vi "Switch Configuration.vi"(8 "error in (no error)":errorcluster, 11 "Node Ptr":T2 format="%.0x") -> (0 "error out":errorcluster)   [LabVIEW 2015, in "DMM-SWITCH-ScanList System Explorer.lvlib"]
uses:
  DMM-SWITCH-ScanList System Explorer.lvlib
  <vilib>/NI Veristand/Custom Device API/Custom Device Item Ref.ctl
  <instrlib>/niSwitch/niSwitch.LLB/niSwitch Topologies.ctl
  Configuration Controls/Switch Config VI UI Data.ctl
  Configuration Controls/Switch Config VI UI Ctrl Values.ctl
  Configuration Controls/Switch Config VI UI Ctrl References.ctl
  <vilib>/NI Veristand/Custom Device API/Custom Device API.lvlib
panel:
  in  "Switch Resource Name":string
  out "Generated Scan List String":string
  in  "Scan List String":string
  in  "Scan List Automatic/Manual":bool=TRUE
  in  "Connect ab0":bool
  in  "Topology Names":T1="2503/2-Wire 24x1 Mux" caption="topology name"
  in  "Save":bool
  in  "Channels":i32[](listbox)
  in  "Switch Model":string(combo)
  in  "Topology":string(combo)
  in  "Remove All":bool
  in  "Add All":bool
  in  "Selectable Channels":i32[](listbox)
  in  "Remove Channels":bool
  in  "Add Channels":bool
  in  "Header":cluster{"Section Name":string}={"Section Name"="Custom Device Item Settings"}
  in  "Description":string
  in  "Name":string
  in  "Update Scan List":bool
  # "Scan List String"
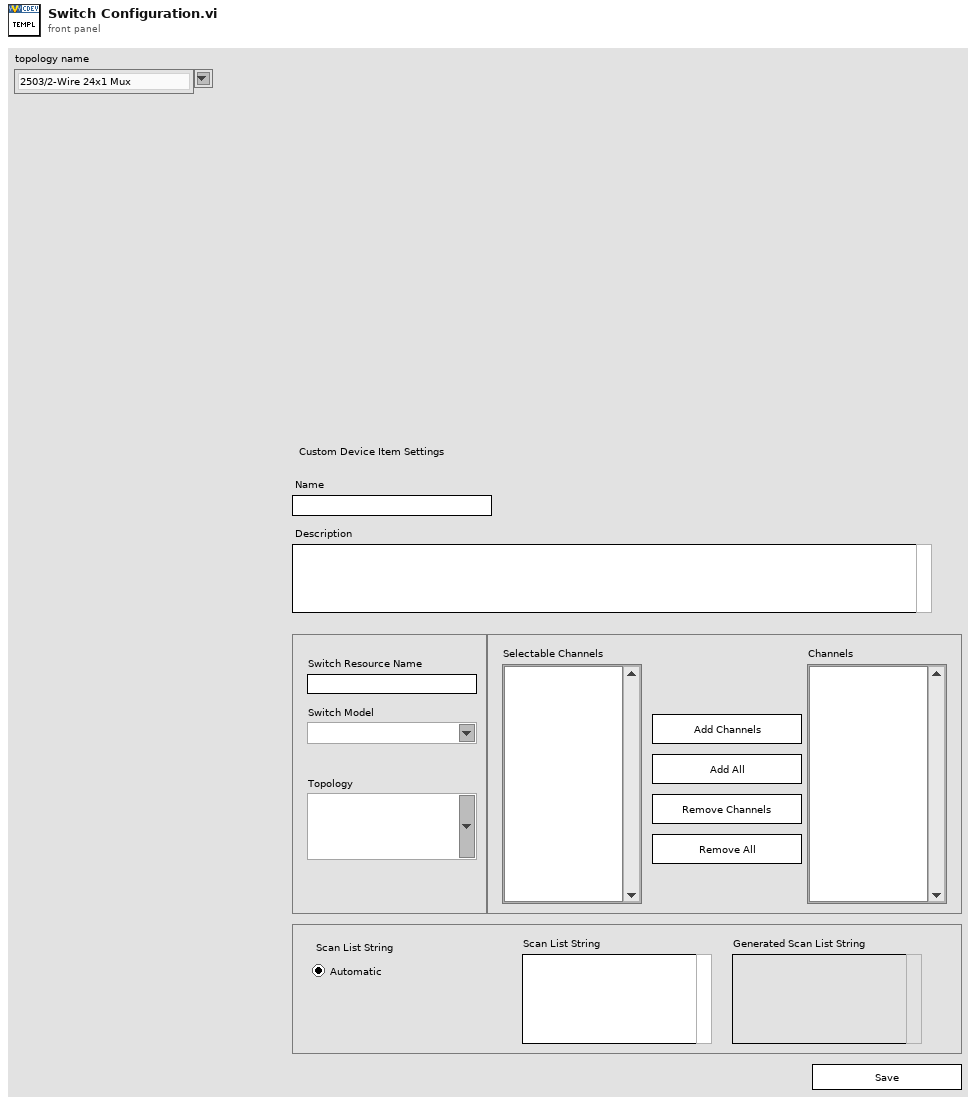
[diagram p1: front panel]
types:
  T1 = typedef "niSwitch Topologies.ctl" = string
  T2 = typedef "Custom Device API.lvlib/Custom Device Item Ref.ctl" = u64
  T3 = typedef "DMM-SWITCH-ScanList System Explorer.lvlib/Switch Config VI UI Data.ctl" = cluster{"Ctrl Values":T4, "Crtl Refs":T5, "Switch Config Page Item Ref":T2, "Mux List":string[]}
  T4 = typedef "DMM-SWITCH-ScanList System Explorer.lvlib/Switch Config VI UI Ctrl Values.ctl" = cluster{"Switch Resource Name":string, "Switch Model":string, "Topology":string, "Selectable Channels":i32[], "Channels":i32[], "Scan List String Mode":bool, "Connect ab0":bool, "Generated Scan List String":string, "Scan List String":string}
  T5 = typedef "DMM-SWITCH-ScanList System Explorer.lvlib/Switch Config VI UI Ctrl References.ctl" = cluster{"Update Scan List":refnum<vi>, "Generated Scan List String":refnum<vi>, "Scan List String":refnum<vi>, "Connect ab0":refnum<vi>, "Selectable Channels":refnum<vi>, "Channels":refnum<vi>, "Topology":refnum<vi>, "Switch Model":refnum<vi>, "Topology Names":refnum<vi>}
  T6 = typedef "Custom Device API.lvlib/Custom Device Item Info.ctl" = cluster{"Name":string, "Is Channel":bool, "GUID":string, "Is Waveform":bool}
  T7 = typedef "Custom Device API.lvlib/Custom Device Commands.ctl" = enum16{"Default", "Item renamed", "Shutdown", "Dynamic button pressed"}
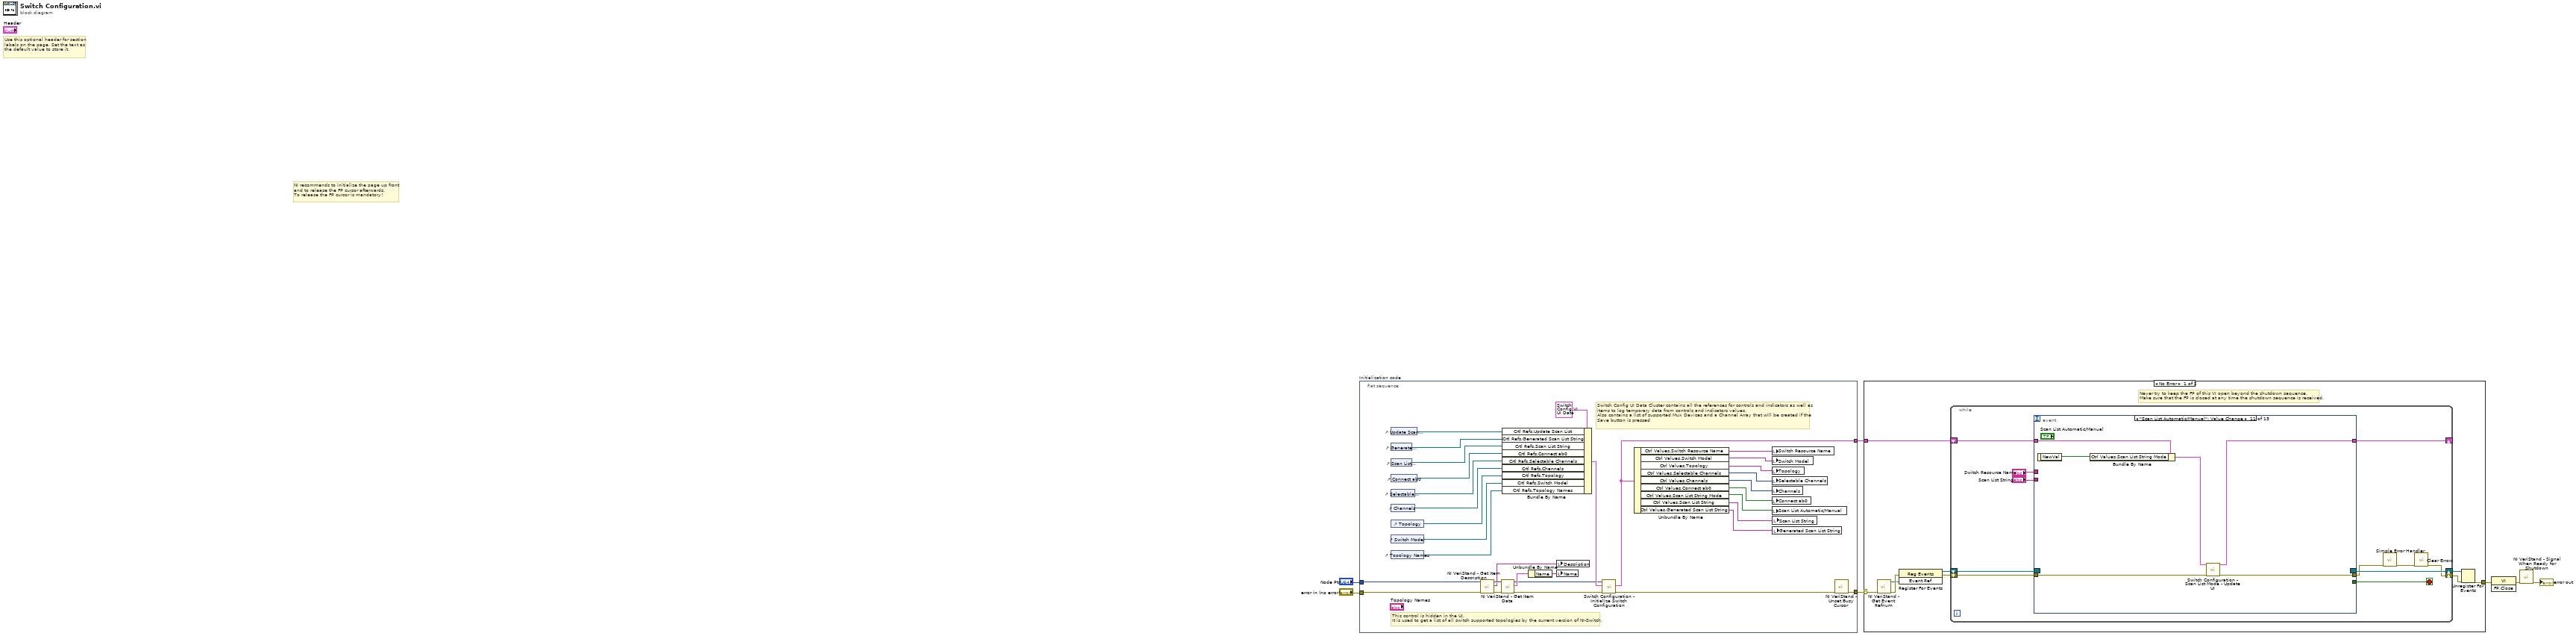
[diagram p0: block diagram]
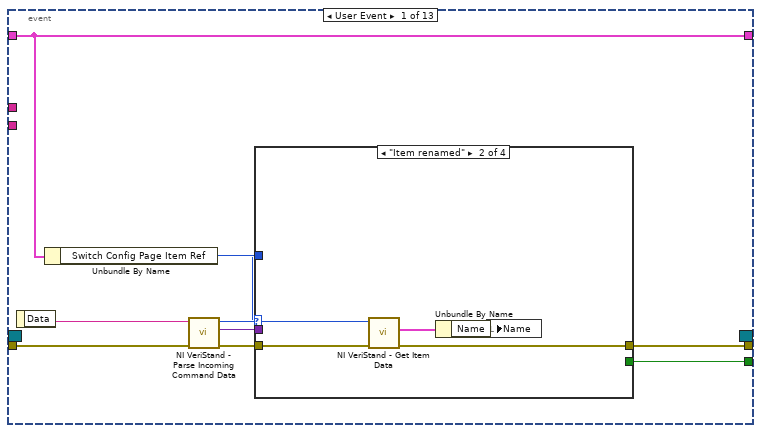
[diagram p2: hidden frame]
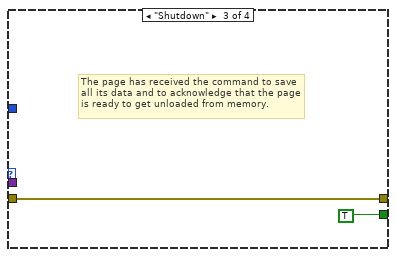
[diagram p4: hidden frame]
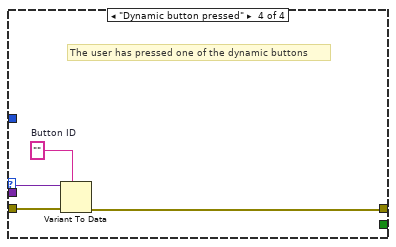
[diagram p5: hidden frame]
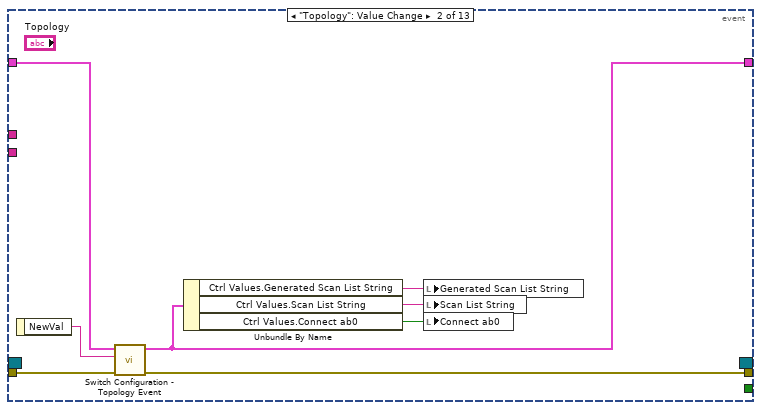
[diagram p6: hidden frame]
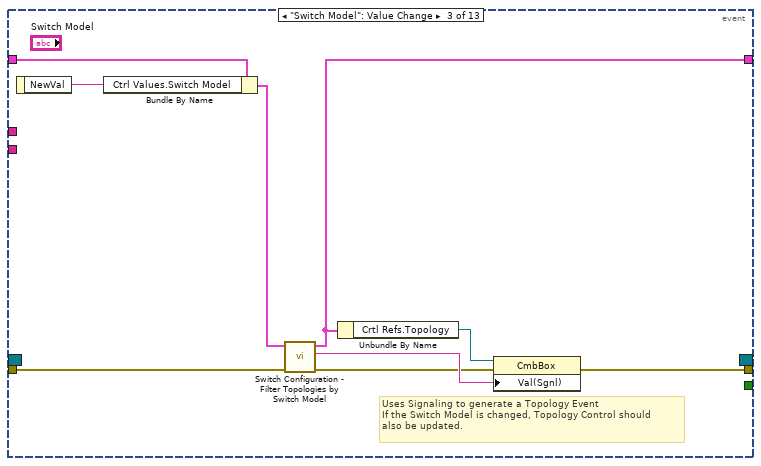
[diagram p7: hidden frame]
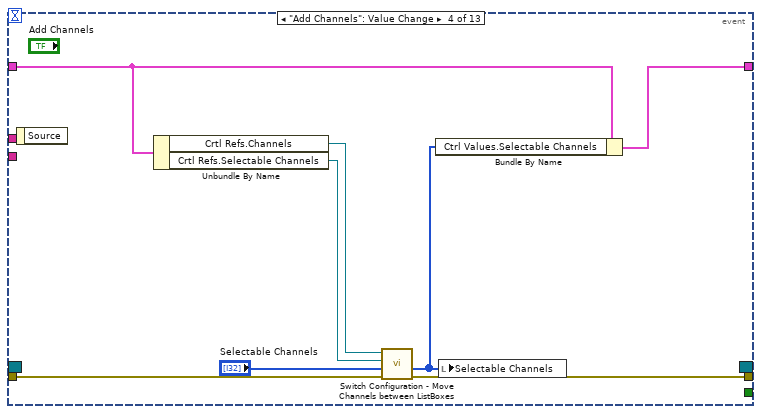
[diagram p8: hidden frame]
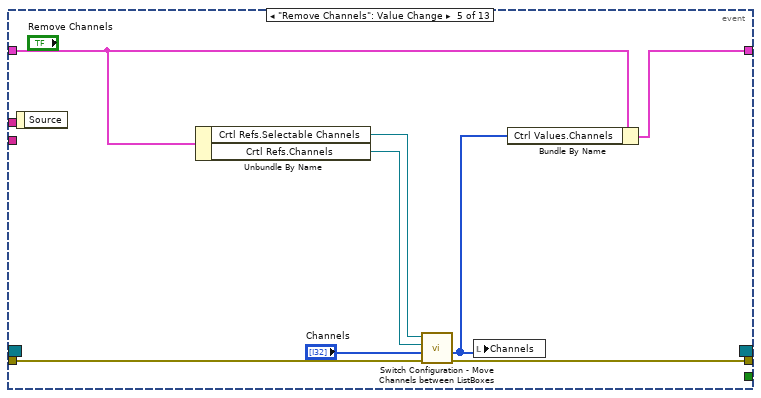
[diagram p9: hidden frame]
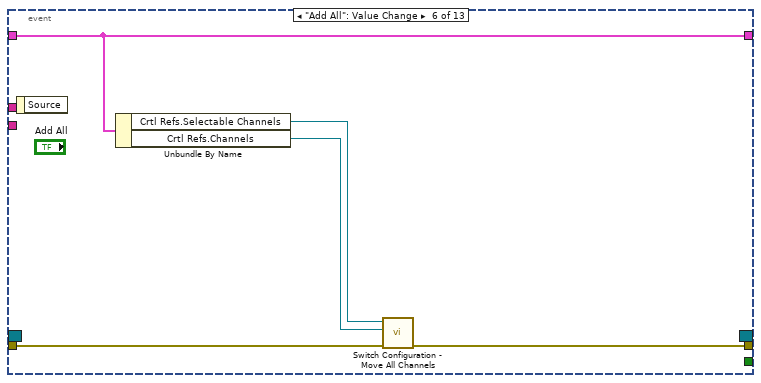
[diagram p10: hidden frame]
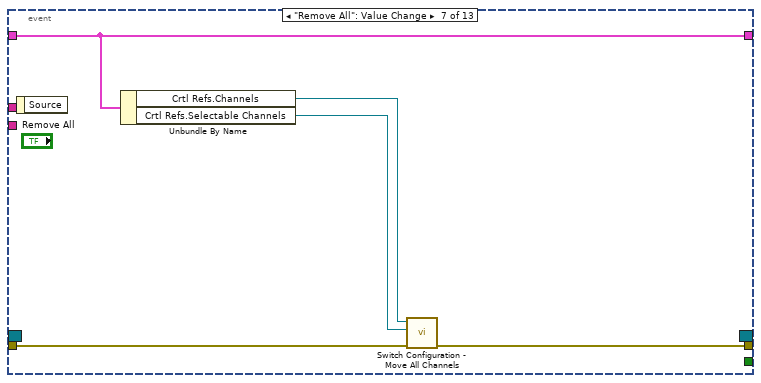
[diagram p11: hidden frame]
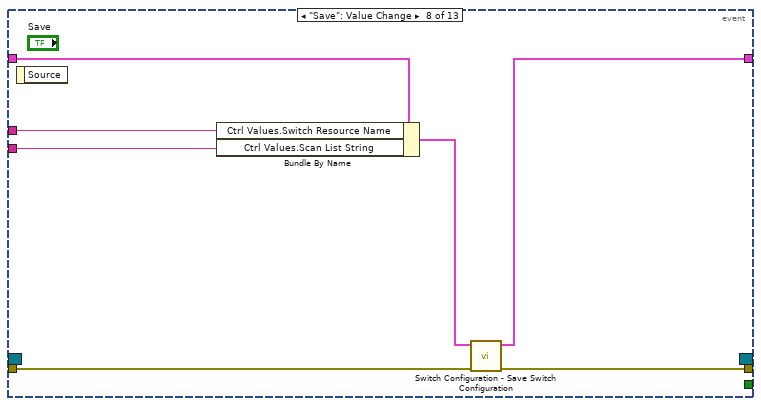
[diagram p12: hidden frame]
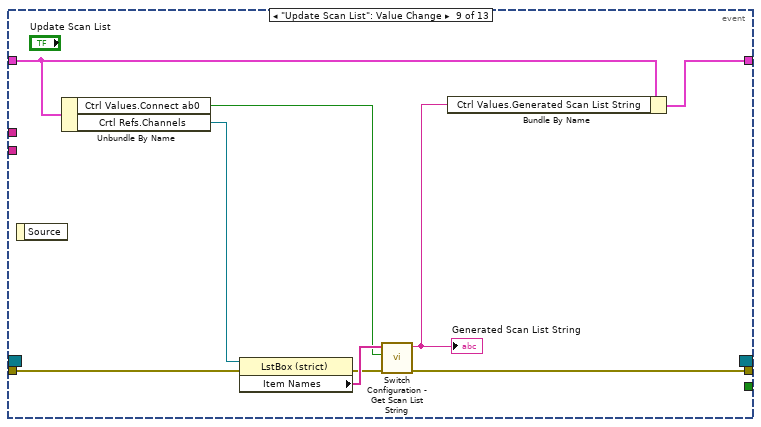
[diagram p13: hidden frame]
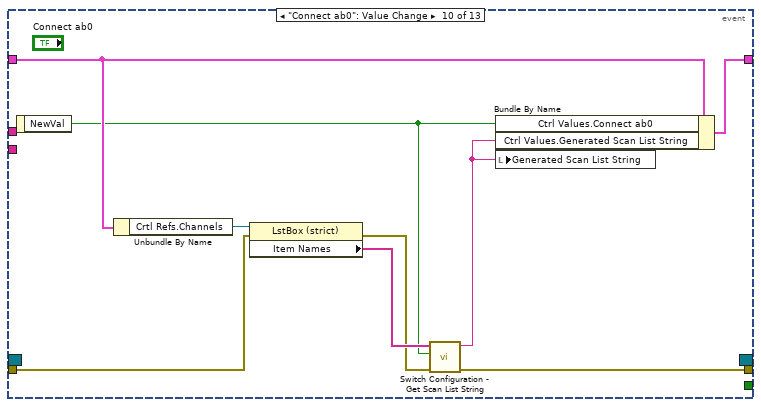
[diagram p14: hidden frame]
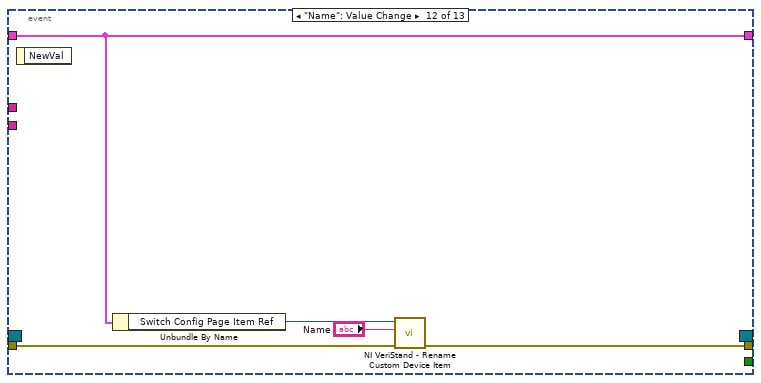
[diagram p15: hidden frame]
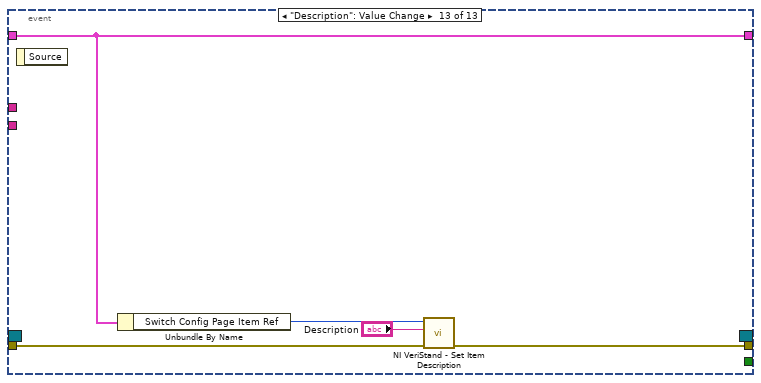
[diagram p16: hidden frame]
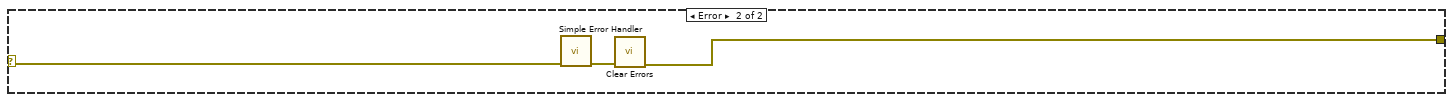
[diagram p17: hidden frame]
diagram:
  # "Use this optional header for section labels on the page. Set the text as the default value to store it."
  # "NI recommends to initialize the page up front\nand to release the FP cursor afterwards.\nTo release the FP cursor is mandatory!"
  n1 = flat-sequence "Initialization code" {
    tunnel: "error in (no error)" -> [w38]
    tunnel: "Node Ptr" -> [w37]
    tunnel: [w20] -> w2
    tunnel: [w10] -> w1
    frame #0 {
      # "This control is hidden in the UI. \nIt is used to get a list of all switch supported topologies by the current version of NI-Switch."
      # "Switch Config UI Data Cluster contains all the references for controls and indicators as well as\nitems to log temporary data from controls and indicators values.\nAlso contains a list of supported Mux Devices and a Channel Array that will be created if the\nSave button is pressed"
      n2 = control-ref of="Update Scan List"() -> (w28:refnum<vi>)
      n3 = control-ref of="Generated Scan List String"() -> (w29:refnum<vi>)
      n4 = control-ref of="Scan List String"() -> (w30:refnum<vi>)
      n5 = control-ref of="Connect ab0"() -> (w31:refnum<vi>)
      n6 = control-ref of="Selectable Channels"() -> (w22:refnum<vi>)
      n7 = control-ref of="Channels"() -> (w23:refnum<vi>)
      n8 = control-ref of="Topology"() -> (w24:refnum<vi>)
      n9 = control-ref of="Switch Model"() -> (w27:refnum<vi>)
      n10 = control-ref of="Topology Names"() -> (w26:refnum<vi>)
      n11 = call <vilib>:"NI VeriStand - Get Item Description.vi"("error in (no error)"=w38, "Item Ref in"=w37) -> ("error out"=w35:errorcluster, "Description"=w36:string, "Item Ref out"=w39:T2)  [unwired: 7 out]
      n12 = call <vilib>:"NI VeriStand - Get Item Data.vi"("error in (no error)"=w35, "Item Ref in"=w39) -> ("error out"=w32:errorcluster, "Item Info"=w34:T6, "Item Ref out"=w9:T2)  [unwired: 7 out]
      n13 = Bundle By Name(cluster=T3 {"Ctrl Values"={"Switch Resource Name"="", "Switch Model"="", "Topology"="", "Selectable Channels"=[], "Channels"=[], "Scan List String Mode"=FALSE, "Connect ab0"=FALSE, "Generated Scan List String"="", "Scan List String"=""}, "Crtl Refs"={"Update Scan List"=refnum, "Generated Scan List String"=refnum, "Scan List String"=refnum, "Connect ab0"=refnum, "Selectable Channels"=refnum, "Channels"=refnum, "Topology"=refnum, "Switch Model"=refnum, "Topology Names"=refnum}, "Switch Config Page Item Ref"=0, "Mux List"=[]} ("Switch Config UI Data"), "Crtl Refs.Update Scan List"=w28, "Crtl Refs.Generated Scan List String"=w29, "Crtl Refs.Scan List String"=w30, "Crtl Refs.Connect ab0"=w31, "Crtl Refs.Selectable Channels"=w22, "Crtl Refs.Channels"=w23, "Crtl Refs.Topology"=w24, "Crtl Refs.Switch Model"=w27, "Crtl Refs.Topology Names"=w26) -> (w21:T3)
      n14 = Unbundle By Name(w34) -> ("Name"=w33:string)
      n15 = local write "Description"(w36) -> ()
      n16 = local write "Name"(w33) -> ()
      n17 = call "Switch Configuration - Initialize Switch Configuration.vi"("error in (no error)"=w32, "Switch Config UI Data in"=w21, "Item Ref in"=w9) -> ("error out"=w8:errorcluster, "Switch Config UI Data out"=w20:T3)  [unwired: 7 in]
      n18 = Unbundle By Name(w20) -> ("Ctrl Values.Switch Resource Name"=w19:string, "Ctrl Values.Switch Model"=w18:string, "Ctrl Values.Topology"=w17:string, "Ctrl Values.Selectable Channels"=w16:i32[], "Ctrl Values.Channels"=w15:i32[], "Ctrl Values.Connect ab0"=w14:bool, "Ctrl Values.Scan List String Mode"=w13:bool, "Ctrl Values.Scan List String"=w12:string, "Ctrl Values.Generated Scan List String"=w11:string)
      n19 = local write "Switch Resource Name"(w19) -> ()
      n20 = local write "Switch Model"(w18) -> ()
      n21 = local write "Topology"(w17) -> ()
      n22 = local write "Selectable Channels"(w16) -> ()
      n23 = local write "Channels"(w15) -> ()
      n24 = local write "Connect ab0"(w14) -> ()
      n25 = local write "Scan List Automatic/Manual"(w13) -> ()
      n26 = local write "Scan List String"(w12) -> ()
      n27 = local write "Generated Scan List String"(w11) -> ()
      n28 = call <vilib>:"NI VeriStand - Unset Busy Cursor.vi"("error in (no error)"=w8) -> ("error out"=w10:errorcluster)  [unwired: 10 out]
    }
  }
  n29 = case shown="No Error" w1 {
    selector: w1 -> [w41 w167]
    tunnel: [w45 w165] -> w7
    tunnel: w2 -> [w40 _]
    frame No Error {
      # "Never try to keep the FP of this VI open beyond the shutdown sequence.\nMake sure that the FP is closed at any time the shutdown sequence is received."
      n30 = call <vilib>:"NI VeriStand - Get Event Refnum.vi"("error in (no error)"=w41) -> ("error out"=w48:errorcluster, "Event Ref"=w44:refnum<user-event>)  [unwired: 9 out]
      n31 = register-events(error in=w48, w44) -> (reference out=w42:refnum<event-registration>, error out=w43:errorcluster)  [unwired: 1 in]
      n32 = while {
        shift-right: [w55] -> w46
        shift-left: w43 -> [w58]
        shift-right: [w59] -> w47
        shift-left: w42 -> [w57]
        shift-right: [w53] -> _
        shift-left: w40 -> [w54]
        stop <- w56 stop-if-true
        n33 = event shown="[10] \"Scan List Automatic/Manual\": Value Change" {
          selector: w57 -> [_ _ _ _ _ _ _ _ _ _ _ _ _]
          dyn-events: [_ _ _ _ _ _ _ _ _ _ _ _ _] -> w59
          timeout: _ -> [_ _ _ _ _ _ _ _ _ _ _ _ _]
          tunnel: w58 -> [w68 w88 w92 w105 w113 w118 w123 w129 w139 w148 w154 w159 w164]
          tunnel: [w64 _ _ _ _ _ _ _ _ _ _ _ _] -> w56
          tunnel: [w63 w87 w95 w103 w111 w117 w122 w130 w136 w145 w153 w158 w163] -> w52
          tunnel: w54 -> [w61 w86 w91 w100 w107 w114 w119 w128 w134 w142 w151 w156 w161]
          tunnel: [w61 w85 w89 w98 w106 w114 w119 w124 w132 w141 w149 w156 w161] -> w53
          tunnel: "Switch Resource Name" -> [_ _ _ _ _ _ _ w127 _ _ _ _ _]
          tunnel: "Scan List String" -> [_ _ _ _ _ _ _ w126 _ _ _ _ _]
          event User Event {
            n34 = event-data() -> ("Data"=w67:string)  [unwired: 1 out]
            n35 = Unbundle By Name(w61) -> ("Switch Config Page Item Ref"=w60:T2)
            n36 = call <vilib>:"NI VeriStand - Parse Incoming Command Data.vi"("error in (no error)"=w68, "Incoming data"=w67) -> ("error out"=w66:errorcluster, "Outgoing data"=w62:variant, "Action"=w65:T7)  [unwired: 7 out]
            n37 = case shown="\"Item renamed\"" w65 {
              tunnel: w66 -> [w69 w74 w75 w80]
              tunnel: [_ _ TRUE _] -> w64
              tunnel: [w69 w71 w75 w77] -> w63
              tunnel: w60 -> [_ w73 _ _]
              tunnel: w62 -> [_ _ _ w79]
              frame "Default", Default {
              }
              frame "Item renamed" {
                n38 = call <vilib>:"NI VeriStand - Get Item Data.vi"("error in (no error)"=w74, "Item Ref in"=w73) -> ("error out"=w71:errorcluster, "Item Info"=w72:T6)  [unwired: 8 out]
                n39 = Unbundle By Name(w72) -> ("Name"=w70:string)
                n40 = local write "Name"(w70) -> ()
              }
              frame "Shutdown" {
                # "The page has received the command to save all its data and to acknowledge that the page is ready to get unloaded from memory."
              }
              frame "Dynamic button pressed" {
                w78 = ""  # Button ID
                # "The user has pressed one of the dynamic buttons"
                n41 = Variant To Data(error in=w80, type=w78, Variant=w79) -> (error out=w77:errorcluster)  [unwired: 1 out]
              }
            }
          }
          event "Topology": Value Change {
            n42 = event-data() -> ("NewVal"=w84:string)  [unwired: 1 out]
            n43 = call "Switch Configuration - Topology Event.vi"("error in (no error)"=w88, "Topology"=w84, "Switch Config UI Data in"=w86) -> ("error out"=w87:errorcluster, "Switch Config UI Data Out"=w85:T3)  [unwired: 7 in]
            n44 = Unbundle By Name(w85) -> ("Ctrl Values.Generated Scan List String"=w83:string, "Ctrl Values.Scan List String"=w82:string, "Ctrl Values.Connect ab0"=w81:bool)
            n45 = local write "Generated Scan List String"(w83) -> ()
            n46 = local write "Scan List String"(w82) -> ()
            n47 = local write "Connect ab0"(w81) -> ()
          }
          event "Switch Model": Value Change {
            # "Uses Signaling to generate a Topology Event\nIf the Switch Model is changed, Topology Control should\nalso be updated."
            n48 = event-data() -> ("NewVal"=w93:string)  [unwired: 1 out]
            n49 = Bundle By Name(cluster=w91, "Ctrl Values.Switch Model"=w93) -> (w90:T3)
            n50 = call "Switch Configuration - Filter Topologies by Switch Model.vi"("error in (no error)"=w92, "Switch Config UI Data In"=w90) -> ("error out"=w96:errorcluster, "First Topology from List"=w97:string, "Switch Config UI Data Out"=w89:T3)  [unwired: 7 in]
            n51 = Unbundle By Name(w89) -> ("Crtl Refs.Topology"=w94:refnum<vi>)
            n52 = property on="Property Node" class="CmbBox"(reference=w94, error in=w96, "Val(Sgnl)"=w97) -> (error out=w95:errorcluster)  [unwired: 1 out]
          }
          event "Add Channels": Value Change {
            n53 = event-data() -> ()  [unwired: 2 out]
            n54 = Unbundle By Name(w100) -> ("Crtl Refs.Channels"=w102:refnum<vi>, "Crtl Refs.Selectable Channels"=w101:refnum<vi>)
            n55 = call "Switch Configuration - Move Channels between ListBoxes.vi"("error in (no error)"=w105, "ListBox Origin In"="Selectable Channels", "ListBox Origin Ref In"=w101, "ListBox Destiny Ref In"=w102) -> ("error out"=w103:errorcluster, "ListBox Out"=w99:i32[])  [unwired: 2 in, 4 out]
            n56 = Bundle By Name(cluster=w100, "Ctrl Values.Selectable Channels"=w99) -> (w98:T3)
            n57 = local write "Selectable Channels"(w99) -> ()
          }
          event "Remove Channels": Value Change {
            n58 = event-data() -> ()  [unwired: 2 out]
            n59 = Unbundle By Name(w107) -> ("Crtl Refs.Selectable Channels"=w110:refnum<vi>, "Crtl Refs.Channels"=w109:refnum<vi>)
            n60 = call "Switch Configuration - Move Channels between ListBoxes.vi"("error in (no error)"=w113, "ListBox Origin In"="Channels", "ListBox Origin Ref In"=w109, "ListBox Destiny Ref In"=w110) -> ("error out"=w111:errorcluster, "ListBox Out"=w108:i32[])  [unwired: 2 in, 4 out]
            n61 = local write "Channels"(w108) -> ()
            n62 = Bundle By Name(cluster=w107, "Ctrl Values.Channels"=w108) -> (w106:T3)
          }
          event "Add All": Value Change {
            n63 = event-data() -> ()  [unwired: 2 out]
            n64 = Unbundle By Name(w114) -> ("Crtl Refs.Selectable Channels"=w116:refnum<vi>, "Crtl Refs.Channels"=w115:refnum<vi>)
            n65 = call "Switch Configuration - Move All Channels.vi"("error in (no error)"=w118, "Destiny Listbox Ref In"=w115, "Origin ListBox Ref In"=w116) -> ("error out"=w117:errorcluster)  [unwired: 4 in, 4 out]
          }
          event "Remove All": Value Change {
            n66 = event-data() -> ()  [unwired: 2 out]
            n67 = Unbundle By Name(w119) -> ("Crtl Refs.Channels"=w121:refnum<vi>, "Crtl Refs.Selectable Channels"=w120:refnum<vi>)
            n68 = call "Switch Configuration - Move All Channels.vi"("error in (no error)"=w123, "Destiny Listbox Ref In"=w120, "Origin ListBox Ref In"=w121) -> ("error out"=w122:errorcluster)  [unwired: 4 in, 4 out]
          }
          event "Save": Value Change {
            n69 = event-data() -> ()  [unwired: 2 out]
            n70 = Bundle By Name(cluster=w128, "Ctrl Values.Switch Resource Name"=w127, "Ctrl Values.Scan List String"=w126) -> (w125:T3)
            n71 = call "Switch Configuration - Save Switch Configuration.vi"("error in (no error)"=w129, "Switch Config UI Data In"=w125) -> ("error out"=w130:errorcluster, "Switch Config UI Data Out"=w124:T3)  [unwired: 8 in]
          }
          event "Update Scan List": Value Change {
            n72 = event-data() -> ()  [unwired: 2 out]
            n73 = Unbundle By Name(w134) -> ("Ctrl Values.Connect ab0"=w131:bool, "Crtl Refs.Channels"=w135:refnum<vi>)
            n74 = property class="LstBox (strict)"(reference=w135, error in=w139) -> (error out=w137:errorcluster, "Item Names"=w138:string[])  [unwired: 1 out]
            n75 = call "Switch Configuration - Get Scan List String.vi"("error in (no error)"=w137, "ab0"=w131, "Channel Array Out"=w138) -> ("error out"=w136:errorcluster, "String"=w133:string)  [unwired: 7 in]
            "Generated Scan List String" <- w133
            n76 = Bundle By Name(cluster=w134, "Ctrl Values.Generated Scan List String"=w133) -> (w132:T3)
          }
          event "Connect ab0": Value Change {
            n77 = event-data() -> ("NewVal"=w140:bool)  [unwired: 1 out]
            n78 = Unbundle By Name(w142) -> ("Crtl Refs.Channels"=w144:refnum<vi>)
            n79 = property class="LstBox (strict)"(reference=w144, error in=w148) -> (error out=w146:errorcluster, "Item Names"=w147:string[])  [unwired: 1 out]
            n80 = call "Switch Configuration - Get Scan List String.vi"("error in (no error)"=w146, "ab0"=w140, "Channel Array Out"=w147) -> ("error out"=w145:errorcluster, "String"=w143:string)  [unwired: 7 in]
            n81 = Bundle By Name(cluster=w142, "Ctrl Values.Connect ab0"=w140, "Ctrl Values.Generated Scan List String"=w143) -> (w141:T3)
            n82 = local write "Generated Scan List String"(w143) -> ()
          }
          event "Scan List Automatic/Manual": Value Change {
            n83 = event-data() -> ("NewVal"=w152:bool)  [unwired: 1 out]
            n84 = Bundle By Name(cluster=w151, "Ctrl Values.Scan List String Mode"=w152) -> (w150:T3)
            n85 = call "Switch Configuration - Scan List Mode - Update UI.vi"("error in (no error)"=w154, "Switch Config UI Data In"=w150) -> ("error out"=w153:errorcluster, "Switch Config UI Data Out"=w149:T3)  [unwired: 8 in]
          }
          event "Name": Value Change {
            n86 = event-data() -> ()  [unwired: 2 out]
            n87 = Unbundle By Name(w156) -> ("Switch Config Page Item Ref"=w155:T2)
            n88 = call <vilib>:"NI VeriStand - Rename Custom Device Item.vi"("error in (no error)"=w159, "New Name"="Name", "Item Ref in"=w155) -> ("error out"=w158:errorcluster)  [unwired: 1 in, 7 out]
          }
          event "Description": Value Change {
            n89 = event-data() -> ()  [unwired: 2 out]
            n90 = Unbundle By Name(w161) -> ("Switch Config Page Item Ref"=w160:T2)
            n91 = call <vilib>:"NI VeriStand - Set Item Description.vi"("error in (no error)"=w164, "Description"="Description", "Item Ref in"=w160) -> ("error out"=w163:errorcluster)  [unwired: 8 out]
          }
        }
        n92 = call <vilib>:"Simple Error Handler.vi"("error in (no error)"=w52) -> ("error out"=w51:errorcluster)  [unwired: 4 in, 4 out]
        n93 = call <vilib>:"Clear Errors.vi"("error in (no error)"=w51) -> ("error out"=w55:errorcluster)  [unwired: 1 in, 5 out]
      }
      n94 = Unregister For Events(event registration refnum=w47, error in=w46) -> (error out=w45:errorcluster)
    }
    frame Error {
      n95 = call <vilib>:"Simple Error Handler.vi"("error in (no error)"=w167) -> ("error out"=w166:errorcluster)  [unwired: 1 in, 7 out]
      n96 = call <vilib>:"Clear Errors.vi"("error in (no error)"=w166) -> ("error out"=w165:errorcluster)  [unwired: 1 in, 5 out]
    }
  }
  n97 = invoke class="VI" method="FP.Close"(error in=w7) -> (error out=w6:errorcluster)  [unwired: 2 in, 2 out]
  n98 = call <vilib>:"NI VeriStand - Signal When Ready for Shutdown.vi"("error in (no error)"=w6) -> ("error out"=→"error out":errorcluster)  [unwired: 10 out]
